vi "Monitoring Page GUID.vi"() -> (3 "Monitoring GUID":string="fc8a3050-8455-4f24-acdb-50198eb01274")   [LabVIEW 2021, in "DSF Shared.lvlib"]
uses:
  DSF Shared.lvlib
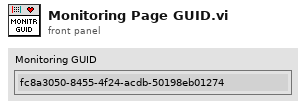
[diagram p1: front panel]
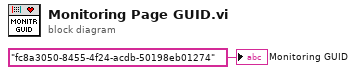
[diagram p0: block diagram]
diagram:
  "Monitoring GUID" <- "fc8a3050-8455-4f24-acdb-50198eb01274" ("Data Sharing Framework")
